vi "20201201 type AB placing error.vi"() -> ()   [LabVIEW 2016]
panel:
  out "Type B rotation error":dbl format="%#_8e"
  out "Type B Y error":dbl format="%#_8g"
  out "Type B X error":dbl format="%#_8g"
  out "Type A rotation error":dbl format="%#_8e"
  out "Type A Y error":dbl format="%#_8g"
  out "Type A X error":dbl format="%#_8g"
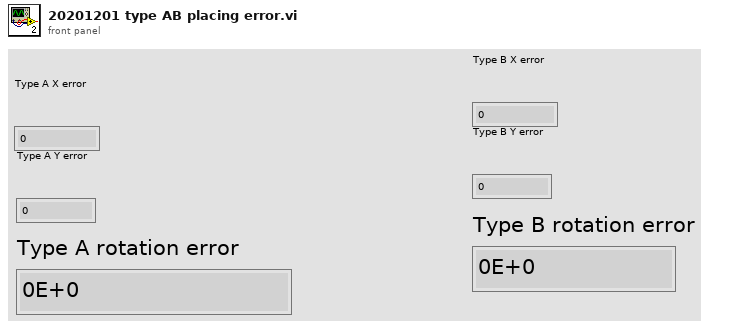
[diagram p1: front panel]
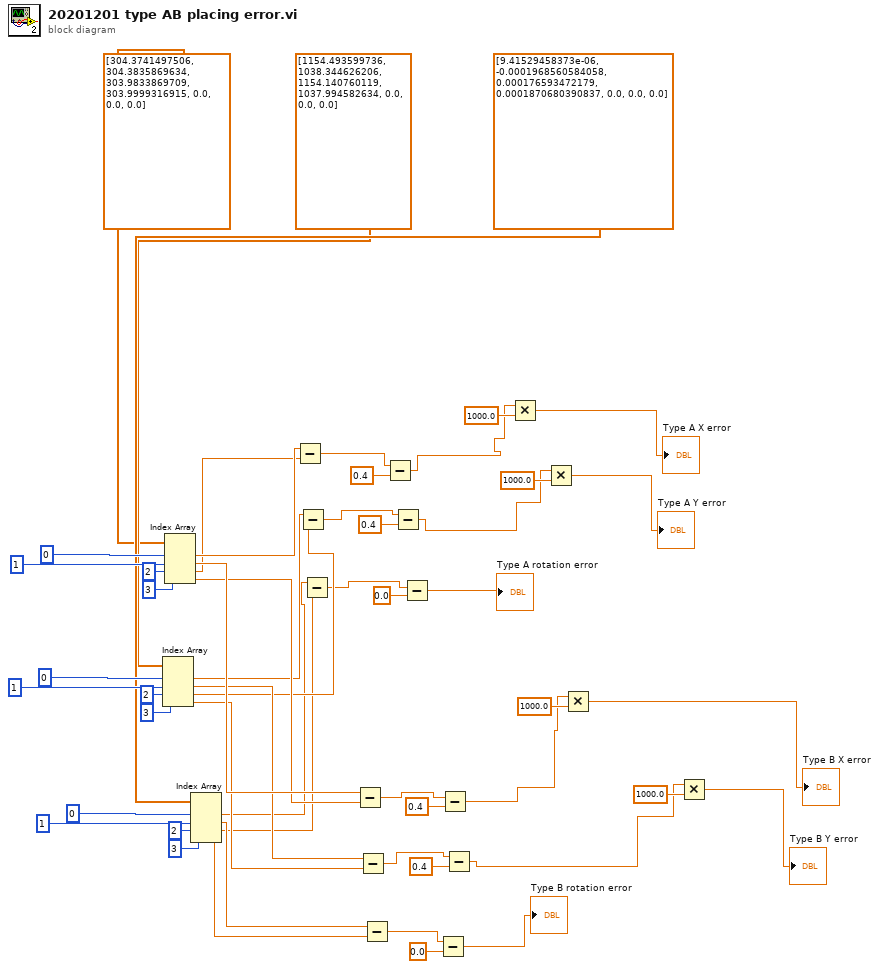
[diagram p0: block diagram]
diagram:
  n1 = Index Array(array=dbl[] [1154.493599736, 1038.344626206, 1154.140760119, 1037.994582634, 0.0, 0.0, 0.0] ("Yposition"), index #1=0 ("index"), index #2=1 ("index"), index #3=2 ("index"), index #4=3 ("index")) -> (element #1=w37:dbl, element #2=w36:dbl, element #3=w35:dbl, element #4=w34:dbl)
  n2 = Index Array(array=dbl[] [304.3741497506, 304.3835869634, 303.9833869709, 303.9999316915, 0.0, 0.0, 0.0] ("X position"), index #1=0 ("index"), index #2=1 ("index"), index #3=2 ("index"), index #4=3 ("index")) -> (element #1=w41:dbl, element #2=w40:dbl, element #3=w39:dbl, element #4=w38:dbl)
  n3 = Index Array(array=dbl[] [9.41529458373e-06, -0.0001968560584058, 0.000176593472179, 0.0001870680390837, 0.0, 0.0, 0.0] ("rotation"), index #1=0 ("index"), index #2=1 ("index"), index #3=2 ("index"), index #4=3 ("index")) -> (element #1=w33:dbl, element #2=w32:dbl, element #3=w31:dbl, element #4=w30:dbl)
  n4 = Subtract(x=w41, y=w39) -> (x-y=w23:dbl)
  n5 = Subtract(x=w37, y=w35) -> (x-y=w22:dbl)
  n6 = Subtract(x=w33, y=w31) -> (x-y=w21:dbl)
  n7 = Subtract(x=w40, y=w38) -> (x-y=w20:dbl)
  n8 = Subtract(x=w36, y=w34) -> (x-y=w19:dbl)
  n9 = Subtract(x=w32, y=w30) -> (x-y=w18:dbl)
  n10 = Subtract(x=w23, y=0.4) -> (x-y=w14:dbl)
  n11 = Subtract(x=w22, y=0.4) -> (x-y=w11:dbl)
  n12 = Subtract(x=w21, y=0.0) -> (x-y=→"Type A rotation error":dbl)
  n13 = Subtract(x=w18, y=0.0) -> (x-y=→"Type B rotation error":dbl)
  n14 = Subtract(x=w20, y=0.4) -> (x-y=w8:dbl)
  n15 = Subtract(x=w19, y=0.4) -> (x-y=w5:dbl)
  n16 = Multiply(x=w14, y=1000.0) -> (x*y=→"Type A X error":dbl)
  n17 = Multiply(x=w11, y=1000.0) -> (x*y=→"Type A Y error":dbl)
  n18 = Multiply(x=w8, y=1000.0) -> (x*y=→"Type B X error":dbl)
  n19 = Multiply(x=w5, y=1000.0) -> (x*y=→"Type B Y error":dbl)
